vi "replace_zero_elements.vi"(10 "array in":cdb[][](array[numeric])) -> (2 "array out":cdb[][](array[numeric]))   [LabVIEW 2010]
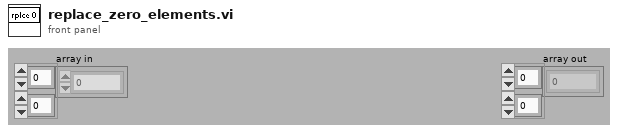
[diagram p1: front panel]
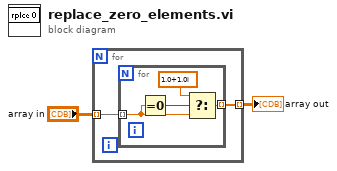
[diagram p0: block diagram]
diagram:
  n1 = for {
    tunnel: "array in" -> [w4] mode=indexing
    tunnel: [w3] -> w1 mode=indexing
    n2 = for {
      tunnel: w4 -> [w6] mode=indexing
      tunnel: [w5] -> w3 mode=indexing
      n3 = Equal To 0?(x=w6) -> (x = 0?=w8:bool)
      n4 = Select(t=cdb 1.0+1.0i, s=w8, f=w6) -> (s? t:f=w5:cdb)
    }
  }
  "array out" <- w1
